vi "Get UID.vi"(8 "error in (no error)":errorcluster, 11 "LV MDI in":refnum<class "LV MDI.lvclass">) -> (0 "error out":errorcluster, 3 "LV MDI out":refnum<class "LV MDI.lvclass">)   [LabVIEW 2016, in "LV MDI.lvclass"]
uses:
  LV MDI.lvclass
  LV MDI.lvclass/LV MDI.ctl
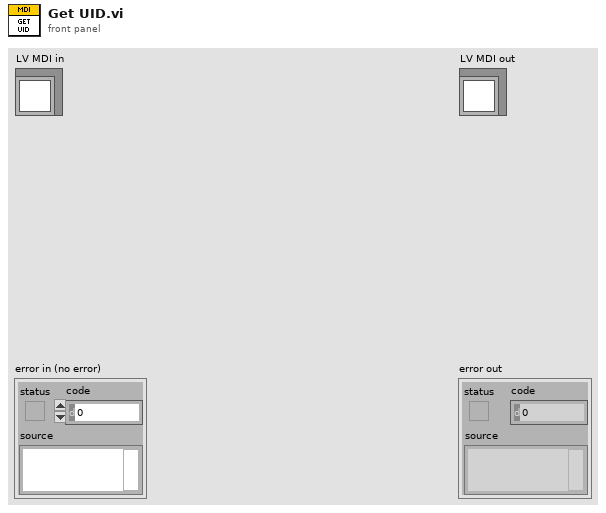
[diagram p1: front panel]
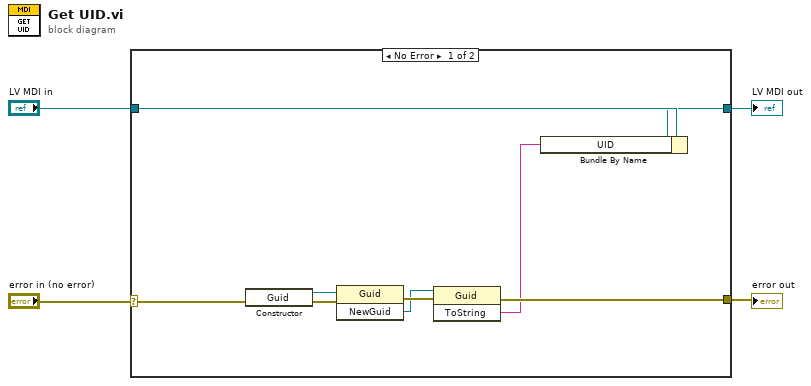
[diagram p0: block diagram]
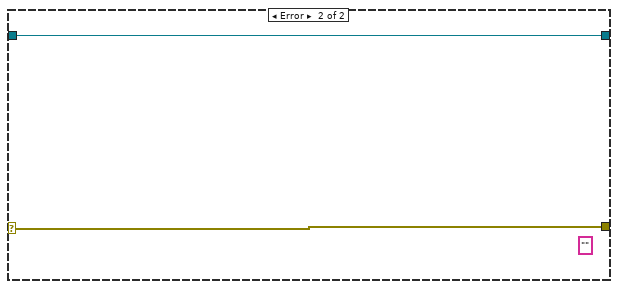
[diagram p2: hidden frame]
diagram:
  n1 = case shown="No Error" "error in (no error)" {
    selector: "error in (no error)" -> [w9 w15]
    tunnel: [w8 w15] -> w3
    tunnel: [w5 w14] -> w1
    tunnel: "LV MDI in" -> [w6 w14]
    frame No Error {
      n2 = constructor class="Guid"(error in=w9) -> (reference out=w10:refnum<k24>, error out=w11:errorcluster)  [unwired: 2 in, 1 out]
      n3 = invoke class="Guid" method="NewGuid"(reference=w10, error in=w11) -> (error out=w13:errorcluster, "NewGuid"=w12:refnum<k24>)  [unwired: 1 in, 1 out]
      n4 = invoke class="Guid" method="ToString"(reference=w12, error in=w13) -> (error out=w8:errorcluster, "ToString"=w7:string)  [unwired: 1 in, 1 out]
      n5 = Bundle By Name(cluster=w6, "UID"=w7) -> (w5:refnum<class "LV MDI.lvclass">)
    }
    frame Error {
      (unwired) "" ("ToString")
    }
  }
  "error out" <- w3
  "LV MDI out" <- w1
